vi "read serial data backup.vi"(8 "error in (no error)":errorcluster, 11 "serial port":refnum<visa-resource-name>) -> (0 "error out":errorcluster, 1 "data read":bool)   [LabVIEW 2017]
uses:
  typedefs/readingType.ctl
  typedefs/reading.ctl
panel:
  out "reading":T1
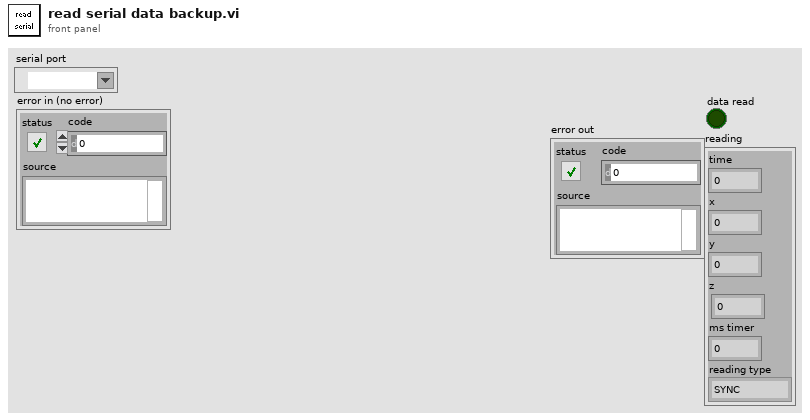
[diagram p1: front panel]
types:
  T1 = typedef "reading.ctl" = cluster{"time":fxp<+,48,48>, "x":sgl, "y":sgl, "z":sgl, "ms timer":u32, "reading type":T2}
  T2 = typedef "readingType.ctl" = enum16{"SYNC", "DETVAL", "COILI", "MAGVEC", "ACCVEC"}
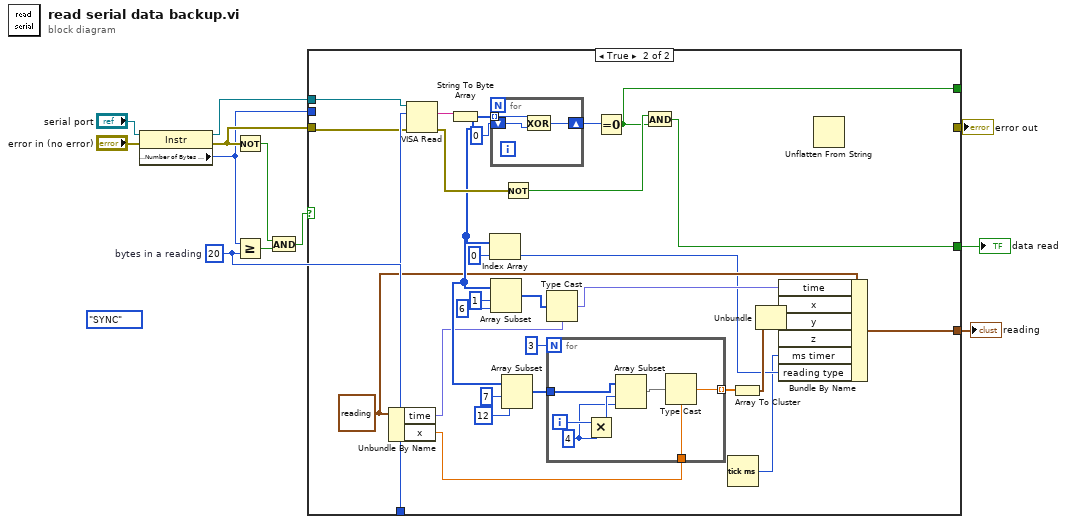
[diagram p0: block diagram]
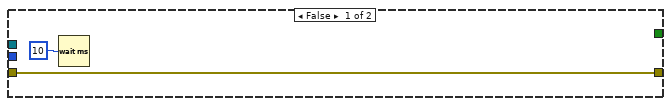
[diagram p2: hidden frame]
diagram:
  (unwired) readingType."SYNC" ("reading type")
  w3 = u32 20  # bytes in a reading
  n1 = property class="Instr"(reference="serial port", error in="error in (no error)") -> (reference out=w12:refnum<visa-resource-name>, error out=w6:errorcluster, "Serial Settings:Number of Bytes at Serial Port"=w4:u32)
  n2 = Not(x=w6) -> (.not. x?=w5:bool)
  n3 = Greater Or Equal?(x=w4, y=w3) -> (x >= y?=w7:bool)
  n4 = And(x=w5, y=w7) -> (x .and. y?=w8:bool)
  n5 = case shown="True" w8 {
    tunnel: w4 -> [_ _]
    tunnel: w12 -> [_ w45]
    tunnel: w6 -> [w14 w43]
    tunnel: [w14 _] -> w9
    tunnel: w3 -> [_ w44]
    tunnel: [_ w37] -> w2
    tunnel: [_ w16] -> w1
    tunnel: [_ w15] -> _
    frame False {
      n6 = Wait (ms)(milliseconds to wait=u32 10) -> ()  [unwired: 1 out]
    }
    frame True {
      w26 = T1 {"time"=0.0, "x"=0.0, "y"=0.0, "z"=0.0, "ms timer"=0, "reading type"=enum."SYNC"} ("reading")
      n7 = Unbundle By Name(w26) -> ("time"=w28:fxp<+,48,48>, "x"=w24:sgl)
      n8 = VISA Read(VISA resource name=w45, byte count=w44, error in (no error)=w43) -> (read buffer=w42:string, error out=w39:errorcluster)  [unwired: 2 out]
      n9 = String To Byte Array(string=w42) -> (unsigned byte array=w33:u8[])
      n10 = Index Array(array=w33, index=0) -> (element=w18:u8)
      n11 = for {
        tunnel: w33 -> [w55] mode=indexing
        shift-right: [w53] -> w40
        shift-left: u8 0 ("y") -> [w54]
        n12 = Exclusive Or(1:w54, 2:w55) -> (0:w53:u8)
      }
      n13 = Array Subset(array=w33, index=1, length=6) -> (w27:u8[])
      n14 = Array Subset(array=w33, index=7, length=12) -> (w30:u8[])
      n15 = Not(x=w39) -> (.not. x?=w38:bool)
      n16 = Type Cast(type=w28, x=w27) -> (*(type *) &x=w25:fxp<+,48,48>)
      n17 = for {
        N: 3 -> [_]
        tunnel: w30 -> [w51]
        tunnel: w24 -> [w47]
        tunnel: [w46] -> w23 mode=indexing
        i -> [w52]
        w49 = 4 ("y")
        n18 = Multiply(x=w52, y=w49) -> (x*y=w50:i32)
        n19 = Array Subset(array=w51, index=w50, length=w49) -> (w48:u8[])
        n20 = Type Cast(type=w47, x=w48) -> (*(type *) &x=w46:sgl)
      }
      n21 = Equal To 0?(x=w40) -> (x = 0?=w15:bool)
      n22 = And(x=w38, y=w15) -> (x .and. y?=w37:bool)
      n23 = Tick Count (ms)() -> (millisecond timer value=w17:u32)
      n24 = Array To Cluster(array=w23) -> (cluster=w22:cluster{"[0]":sgl, "[1]":sgl, "[2]":sgl})
      n25 = Unbundle(w22) -> ("[0]"=w21:sgl, "[1]"=w20:sgl, "[2]"=w19:sgl)
      n26 = Bundle By Name(cluster=w26, "time"=w25, "x"=w21, "y"=w20, "z"=w19, "ms timer"=w17, "reading type"=w18) -> (w16:T1)
      n27 = Unflatten From String() -> ()  [unwired: 5 in, 3 out]
    }
  }
  "error out" <- w9
  "data read" <- w2
  "reading" <- w1
